vi "OpenCloseTreeItem.vi"(8 "error in (no error)":errorcluster, 9 "Open?":bool, 10 "Item Tag in":string, 11 "TreeControl in":refnum<vi>) -> (0 "error out":errorcluster, 2 "Item Tag out":string, 3 "TreeControl out":refnum<vi>)   [LabVIEW 2018]
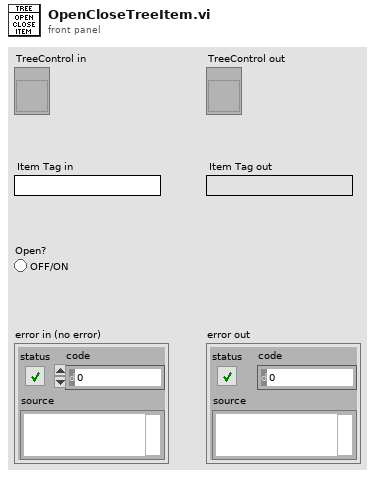
[diagram p1: front panel]
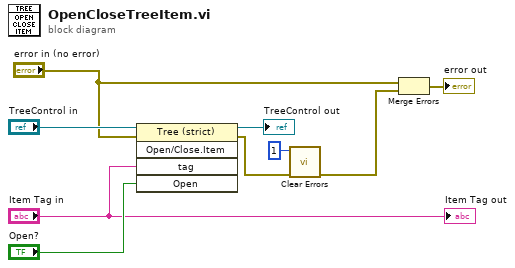
[diagram p0: block diagram]
diagram:
  n1 = invoke class="Tree (strict)" method="Open/Close.Item"(reference="TreeControl in", error in="error in (no error)", "tag"="Item Tag in", "Open"="Open?") -> (reference out=→"TreeControl out":refnum<vi>, error out=w5:errorcluster)  [unwired: 1 in, 3 out]
  n2 = call <vilib>:"Clear Errors.vi"("error in (no error)"=w5, "specific error code to clear (0: all)"=1) -> ("error out"=w2:errorcluster)  [unwired: 4 in, 1 out]
  n3 = Merge Errors("error in (no error)", w2) -> (→"error out":errorcluster)
  "Item Tag out" <- "Item Tag in"
